vi "move_stage_to_target_seq.vi"(10 "event":T1=enum."stage.MoveTo1", 11 "Stage events":refnum<queue>) -> ()   [LabVIEW 2012]
uses:
  typedefs/StageEvent.ctl
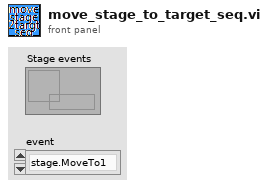
[diagram p1: front panel]
types:
  T1 = typedef "StageEvent.ctl" = enum16{"stage.TimeOut", "stage.FlushData", "stage.GetPosition", "stage.Init", "stage.MoveTo1", "stage.MoveTo2", "stage.MoveTo3", "stage.Stop"}
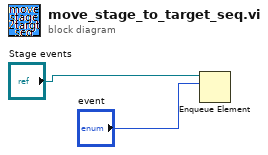
[diagram p0: block diagram]
diagram:
  n1 = Enqueue Element(queue="Stage events", element="event") -> ()  [unwired: 2 in, 3 out]
